vi "From Pythonic - String.vi"(4 "Pythonic Value":string) -> (1 "String":string)   [LabVIEW 2012, in "OPI.lvclass"]
doc: "Convert pythonic values into LabVIEW data. This method can be helpfull to convert elements of tuples or dictionaries.\n\nReturn a string."
uses:
  OPI.lvclass
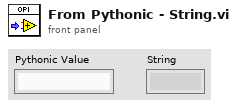
[diagram p1: front panel]
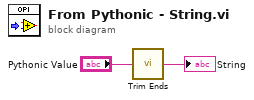
[diagram p0: block diagram]
diagram:
  n1 = call "Trim Ends.vi"("String"="Pythonic Value") -> ("Trimmed String"=→"String":string)
